vi "FPGA_ReadAnalogTriggerOutput.vi"(8 "error in (no error)":errorcluster, 11 "AnalogTriggerDevRef":T1) -> (0 "error out":errorcluster, 1 "Trigger State":bool, 2 "In Window":bool, 3 "AnalogTriggerDevRef":T1)   [LabVIEW 2017]
uses:
  <vilib>/Rock Robotics/SystemInterfaces/AnalogTrigger/FPGA_AnalogTriggerDevRef.ctl
  <vilib>/Rock Robotics/SystemInterfaces/AnalogTrigger/FPGA_AnalogTriggerIndex.ctl
  <vilib>/Rock Robotics/SystemInterfaces/System/FPGA_SystemFPGA Ref Global.vi
  <vilib>/Utility/error.llb/Error Cluster From Error Code.vi
  <vilib>/rvi/errors/niLvFpgaAdjustHostInterfaceError.vi
  <vilib>/rvi/interface/nirviReadWriteControl/nirviReadWriteControl.xnode
  <vilib>/Rock Robotics/SystemInterfaces/System/FPGA_SystemFRC FPGA Ref.ctl
  NiFpgaLv.dll
  <vilib>/rvi/interface/Simulation/niFpgaSimulationCallBeginRW.vi
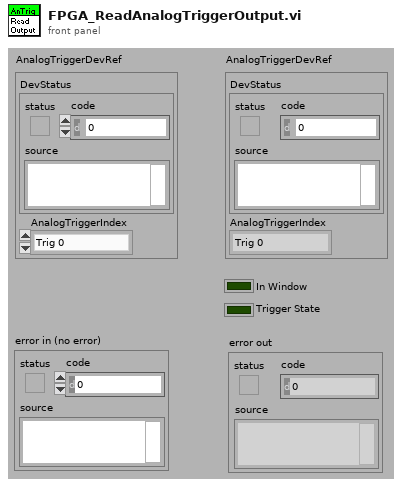
[diagram p1: front panel]
types:
  T1 = typedef "FPGA_AnalogTriggerDevRef.ctl" = cluster{"DevStatus":errorcluster, "AnalogTriggerIndex":T2}
  T2 = typedef "FPGA_AnalogTriggerIndex.ctl" = enum8{"Trig 0", "Trig 1", "Trig 2", "Trig 3", "Trig 4", "Trig 5", "Trig 6", "Trig 7", "Invalid"}
  T3 = typedef "FPGA_SystemFRC FPGA Ref.ctl" = refnum<k20>
  T4 = cluster{"InHysteresis":bool, "OverLimit":bool, "Rising":bool, "Falling":bool}[]
  T5 = cluster{"InHysteresis":bool, "OverLimit":bool, "Rising":bool, "Falling":bool}
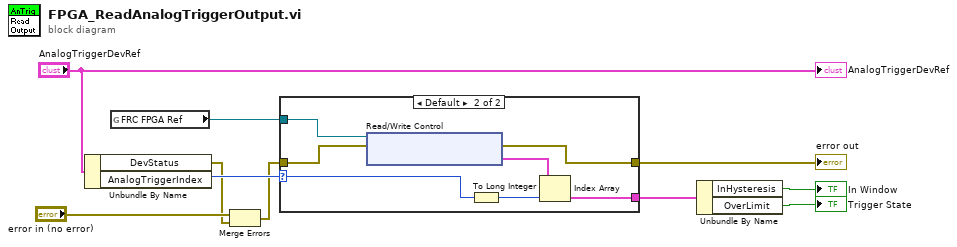
[diagram p0: block diagram]
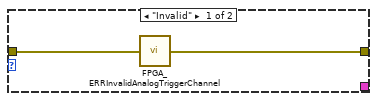
[diagram p2: hidden frame]
diagram:
  n1 = Unbundle By Name("AnalogTriggerDevRef") -> ("DevStatus"=w4:errorcluster, "AnalogTriggerIndex"=w7:T2)
  n2 = global read "FPGA_SystemFPGA Ref Global.vi" "FRC FPGA Ref"() -> (w6:T3)
  n3 = Merge Errors("error in (no error)", w4) -> (w3:errorcluster)
  n4 = case shown="Default" w7 {
    selector: w7 -> [_ w18]
    tunnel: w3 -> [w12 w14]
    tunnel: [w11 w19] -> w10
    tunnel: [_ w17] -> w2
    tunnel: w6 -> [_ w15]
    frame "Invalid" {
      n5 = call <vilib>:"FPGA_ERRInvalidAnalogTriggerChannel.vi"("error in (no error)"=w12) -> ("error out"=w11:errorcluster)
    }
    frame Default {
      n6 = xnode "Read/Write Control"("FPGA VI Reference In"=w15, "error in"=w14) -> ("error out"=w19:errorcluster, "AnalogTrigger.Output"=w13:T4)  [unwired: 1 out]
      n7 = To Long Integer(number=w18) -> (32bit integer=w16:i32)
      n8 = Index Array(array=w13, index=w16) -> (element=w17:T5)
    }
  }
  "error out" <- w10
  n9 = Unbundle By Name(w2) -> ("InHysteresis"=→"In Window":bool, "OverLimit"=→"Trigger State":bool)
  "AnalogTriggerDevRef" <- "AnalogTriggerDevRef"
